vi "Pfeiffer-RVC300.contents.vi"() -> ()   [LabVIEW 2014, in "Pfeiffer-RVC300.lvlib"]
doc: "loads all VIs into memory - required for building an application"
uses:
  Pfeiffer-RVC300.lvlib
panel:
  out "error out":errorcluster
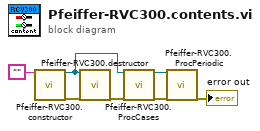
[diagram p0: block diagram]
diagram:
  n1 = call "Pfeiffer-RVC300.constructor.vi"("name"="") -> ("i ref out"=w7:refnum<vi>, "error out"=w3:errorcluster)  [unwired: 16 in, 1 out]
  n2 = call "Pfeiffer-RVC300.destructor.vi"("i ref in"=w7, "error in(no error)"=w3) -> ("error out"=w4:errorcluster)  [unwired: 17 in]
  n3 = call "Pfeiffer-RVC300.ProcCases.vi"("i ref in"=w7, "error in (no error)"=w4) -> ("i ref out"=w6:refnum<vi>, "error out"=w5:errorcluster)  [unwired: 15 in, 1 out]
  n4 = call "Pfeiffer-RVC300.ProcPeriodic.vi"("i ref in"=w6, "error in (no error)"=w5) -> ("error out"=→"error out":errorcluster)  [unwired: 15 in, 2 out]
